vi "Read Is quiet.vi"(11 "CDependencyInspection in":refnum<class "CDependencyInspection.lvclass">) -> (2 "quiet?":bool, 3 "CDependencyInspection out":refnum<class "CDependencyInspection.lvclass">)   [LabVIEW 2020, in "DependencyInspection.lvlib" / "CDependencyInspection.lvclass"]
uses:
  CDependencyInspection.lvclass
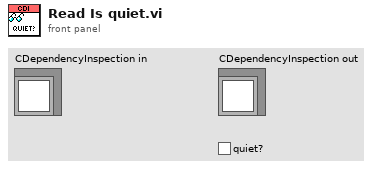
[diagram p1: front panel]
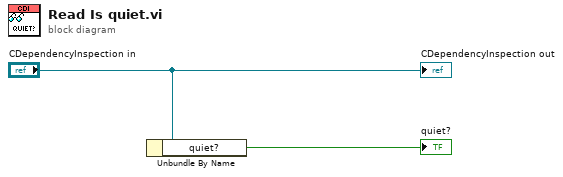
[diagram p0: block diagram]
diagram:
  n1 = Unbundle By Name("CDependencyInspection in") -> ("quiet?"=→"quiet?":bool)
  "CDependencyInspection out" <- "CDependencyInspection in"
